vi "Create.vi"(8 "error in (no error)":errorcluster, 10 "Digital Configuration Parameters":T1) -> (0 "error out":errorcluster, 3 "Digital Output out":refnum<class "Digital Output.lvclass">)   [LabVIEW 2021, in "Digital Output.lvlib" / "Digital Output.lvclass"]
uses:
  Digital Output.lvclass
  Digital Output.lvclass/Digital Output.ctl
  <resource>/objmgr/daqmx.rc
  <vilib>/DAQmx/write.llb/DAQmx Write (Digital Bool 1Line 1Point).vi
  <vilib>/DAQmx/create/channels.llb/DAQmx Create Channel (DO-Digital Output).vi
  Utilities/Digital Configuration Parameters.ctl
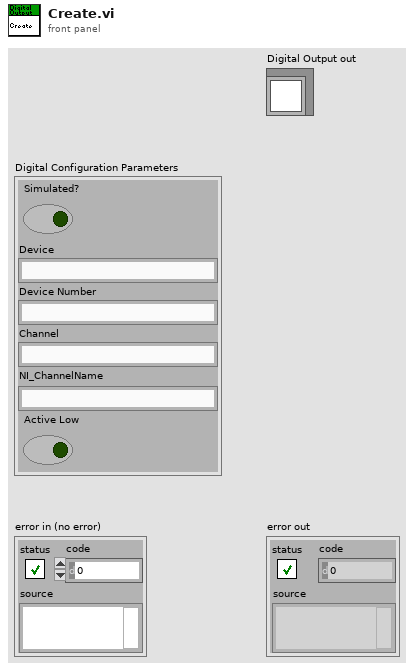
[diagram p1: front panel]
types:
  T1 = typedef "Digital Configuration Parameters.ctl" = cluster{"Simulated?":bool, "Device":string, "Device Number":string, "Channel":string, "NI_ChannelName":string, "Active Low":bool}
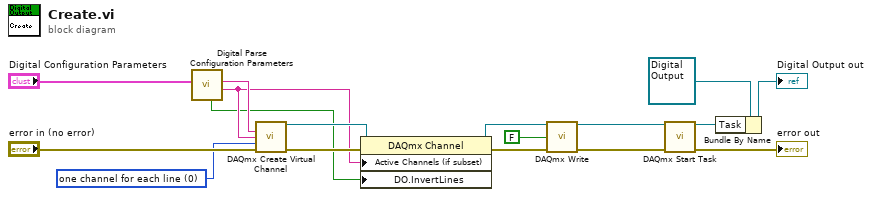
[diagram p0: block diagram]
diagram:
  w1 = 0 items=["one channel for each line", "one channel for all lines"] ("line grouping")
  n1 = call "Digital Parse Configuration Parameters.vi"("Digital Configuration Parameters"="Digital Configuration Parameters") -> ("name to assign"=w4:string, "lines"=w5:string, "Active Low"=w3:bool)  [unwired: 8 in]
  n2 = call-poly <vilib>:"DAQmx Create Virtual Channel.vi"("lines"=w5, "name to assign"=w4, "line grouping"=w1, "error in"="error in (no error)") -> ("task out"=w17:refnum<k21>, "error out"=w16:errorcluster)  [unwired: 10 in]
  n3 = property class="DAQmx Channel"(reference=w17, error in=w16, "Active Channels (if subset)"=w4, "DO.InvertLines"=w3) -> (reference out=w12:refnum<k21>, error out=w11:errorcluster)
  n4 = call-poly <vilib>:"DAQmx Write.vi"("task/channels in"=w12, "data"=FALSE, "error in"=w11) -> ("task out"=w14:refnum<k21>, "error out"=w13:errorcluster)  [unwired: 10 in, 1 out]
  n5 = call <vilib>:"DAQmx Start Task.vi"("task/channels in"=w14, "error in"=w13) -> ("task out"=w15:refnum<k21>, "error out"=→"error out":errorcluster)  [unwired: 12 in]
  n6 = Bundle By Name(cluster=refnum<class "Digital Output.lvclass"> refnum ("Digital Output out"), "Task"=w15) -> (→"Digital Output out":refnum<class "Digital Output.lvclass">)
